vi "CLC_CMD_Module_Query.vi"(7 "CMD in":string, 8 "error in":errorcluster, 11 "TCPIPin":T1={"address"="192.168.100.111", "remote port or service name"=5025, "timeout ms (60000)"=10000}) -> (0 "error out":errorcluster, 2 "data out":string, 3 "TCPIPout":T1={"address"="192.168.100.111", "remote port or service name"=5025, "timeout ms (60000)"=10000})   [LabVIEW 2023]
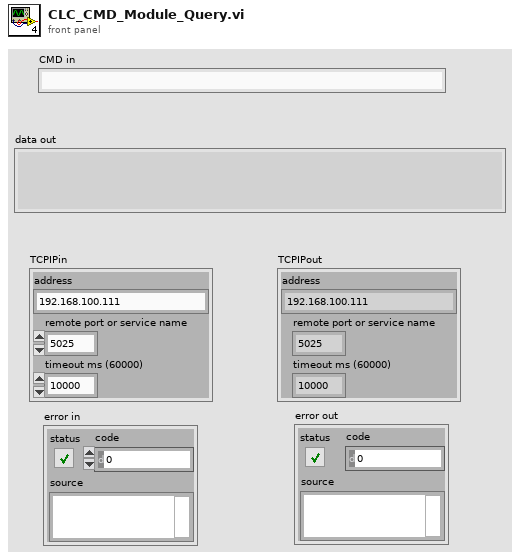
[diagram p1: front panel]
types:
  T1 = cluster{"address":string, "remote port or service name":u16, "timeout ms (60000)":i32}
  T2 = enum16{"Standard", "Buffered", "CRLF", "Immediate"}
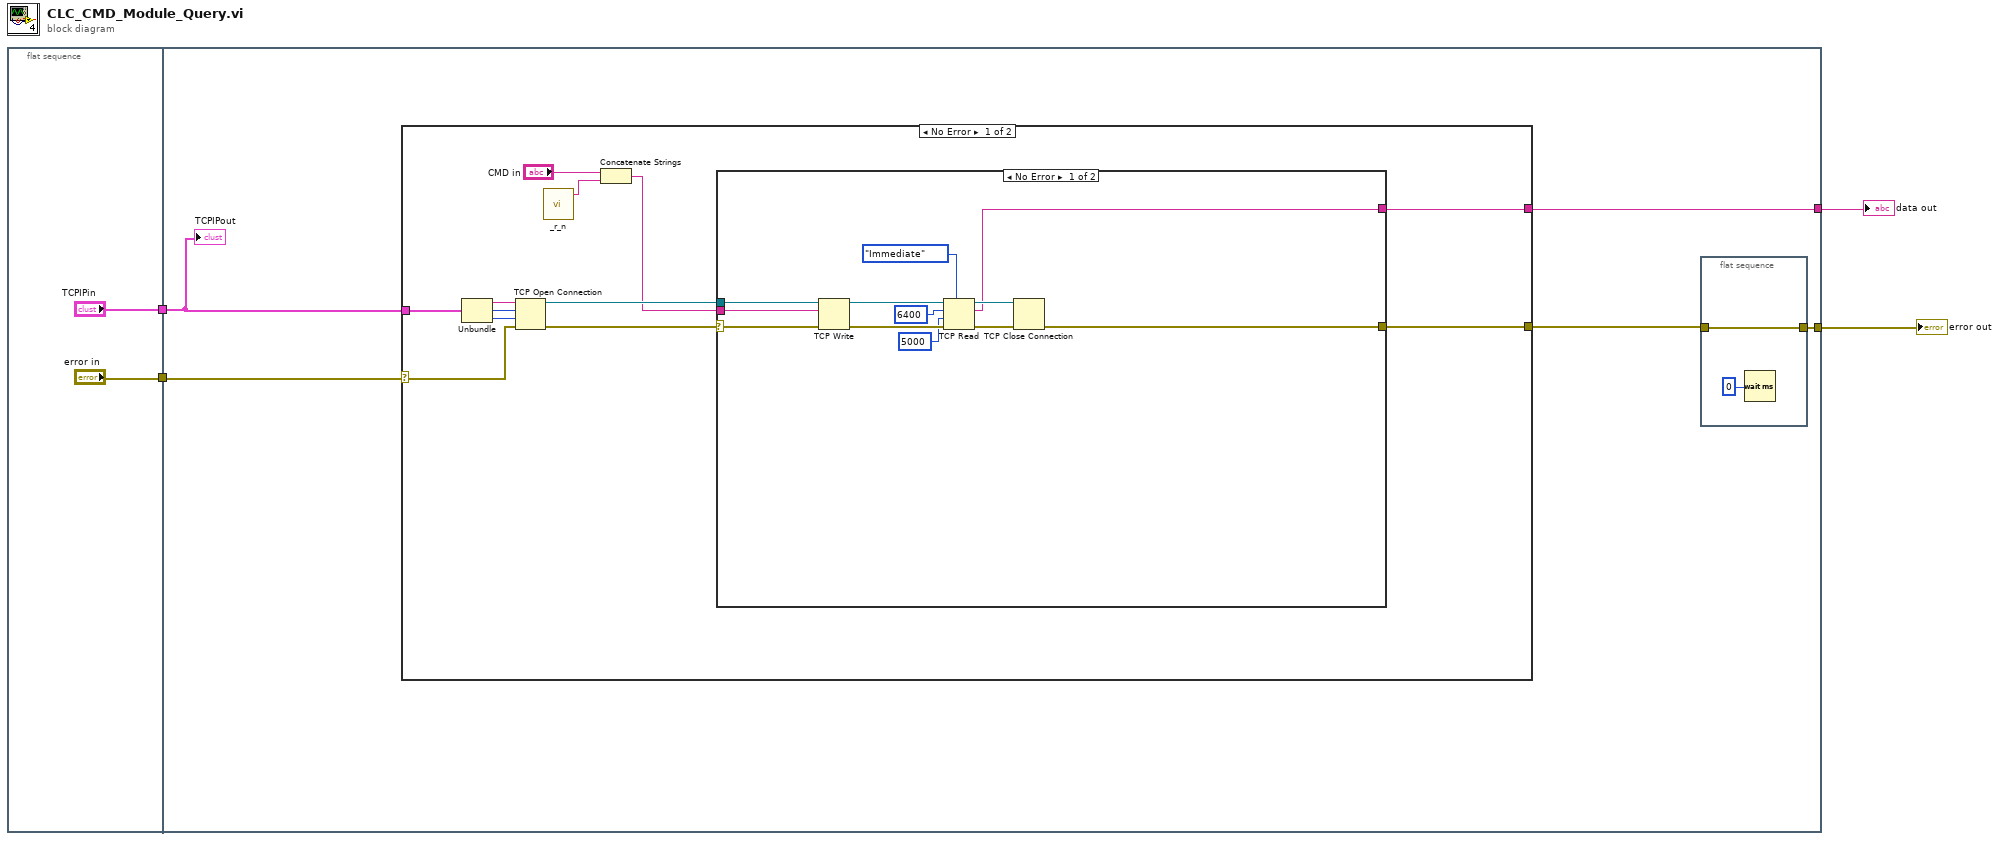
[diagram p0: block diagram]
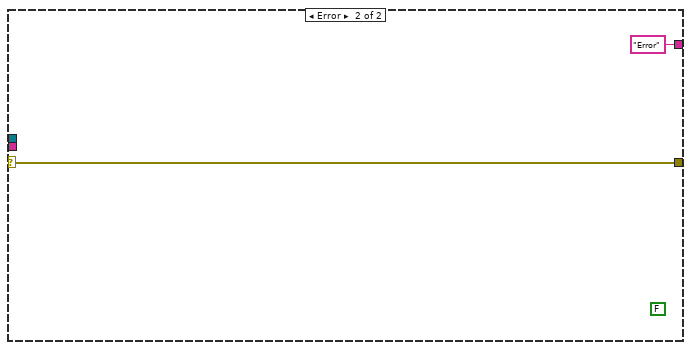
[diagram p2: hidden frame]
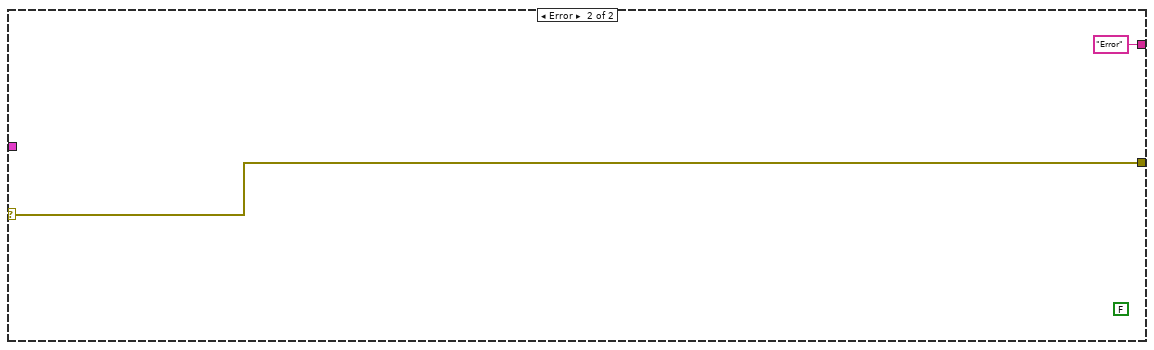
[diagram p3: hidden frame]
diagram:
  n1 = flat-sequence {
    tunnel: ["TCPIPin"] -> w4
    tunnel: ["error in"] -> w3
    tunnel: w4 -> [w11]
    tunnel: w3 -> [w9]
    tunnel: [w10] -> w2
    tunnel: [w8] -> w1
    frame #0 {
    }
    frame #1 {
      n2 = case shown="No Error" w9 {
        selector: w9 -> [w16 w39]
        tunnel: w11 -> [w17 _]
        tunnel: [w15 "Error" ("data out")] -> w8
        tunnel: [w22 w39] -> w7
        frame No Error {
          n3 = Unbundle(w17) -> ("address"=w19:string, "remote port or service name"=w20:u16, "timeout ms (60000)"=w21:i32)
          n4 = TCP Open Connection(address=w19, remote port or service name=w20, timeout ms (60000)=w21, error in (no error)=w16) -> (connection ID=w18:refnum<k5>, error out=w14:errorcluster)  [unwired: 1 in]
          n5 = call "_r_n.vi"() -> ("command"=w12:string)  [unwired: 5 in]
          n6 = Concatenate Strings("CMD in", w12) -> (w13:string)
          n7 = case shown="No Error" w14 {
            selector: w14 -> [w24 w37]
            tunnel: w13 -> [w35 _]
            tunnel: [w34 w37] -> w22
            tunnel: w18 -> [w29 _]
            tunnel: [w25 "Error" ("data out")] -> w15
            frame No Error {
              n8 = TCP Write(connection ID=w29, data in=w35, error in (no error)=w24) -> (connection ID out=w31:refnum<k5>, error out=w30:errorcluster)  [unwired: 1 in, 1 out]
              n9 = TCP Read(connection ID=w31, bytes to read=6400, error in (no error)=w30, 7:T2."Immediate" ("mode (standard)"), 9:5000 ("timeout ms (25000)")) -> (connection ID out=w32:refnum<k5>, data out=w25:string, error out=w33:errorcluster)
              n10 = TCP Close Connection(connection ID=w32, error in (no error)=w33) -> (error out=w34:errorcluster)  [unwired: 1 in, 1 out]
            }
            frame Error {
              (unwired) FALSE
            }
          }
        }
        frame Error {
          (unwired) FALSE
        }
      }
      n11 = flat-sequence {
        tunnel: w7 -> [w41]
        tunnel: [w41] -> w10
        frame #0 {
          n12 = Wait (ms)(milliseconds to wait=u32 0) -> ()  [unwired: 1 out]
        }
      }
      "TCPIPout" <- w11
    }
  }
  "error out" <- w2
  "data out" <- w1
